vi "GDSError_LogErrorInformation.vi"(1 "State":string, 2 "LocalVariableData":variant, 3 "ExtraErrorInfo":string, 5 "error in (no error)":errorcluster) -> (19 "error out":errorcluster)   [LabVIEW 2016]
doc: "You can use this VI to generate errors."
uses:
  <resource>/Framework/Providers/Open_GDS/ClassProviders/Common/Error/GDSError_LogCluster.ctl
  <resource>/Framework/Providers/Open_GDS/ClassProviders/Common/Error/private/GDSError_LogCases.ctl
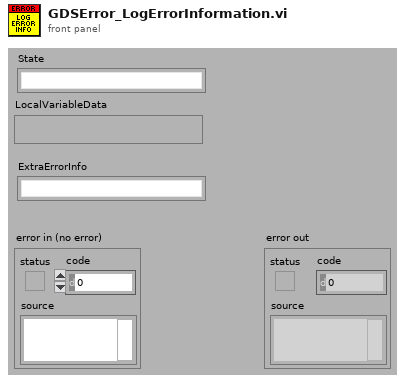
[diagram p1: front panel]
types:
  T1 = typedef "GDSError_LogCases.ctl" = enum16{"Init", "AddError", "ReadFirstError", "ReadLatestError", "ReadAllErrors", "ClearError", "ClearAllErrors"}
  T2 = typedef "GDSError_LogCluster.ctl" = cluster{"Time":timestamp, string, "error IO":errorcluster, "State":string, "LocalVariabelXML":string, "ExtraErrorInfo":string}
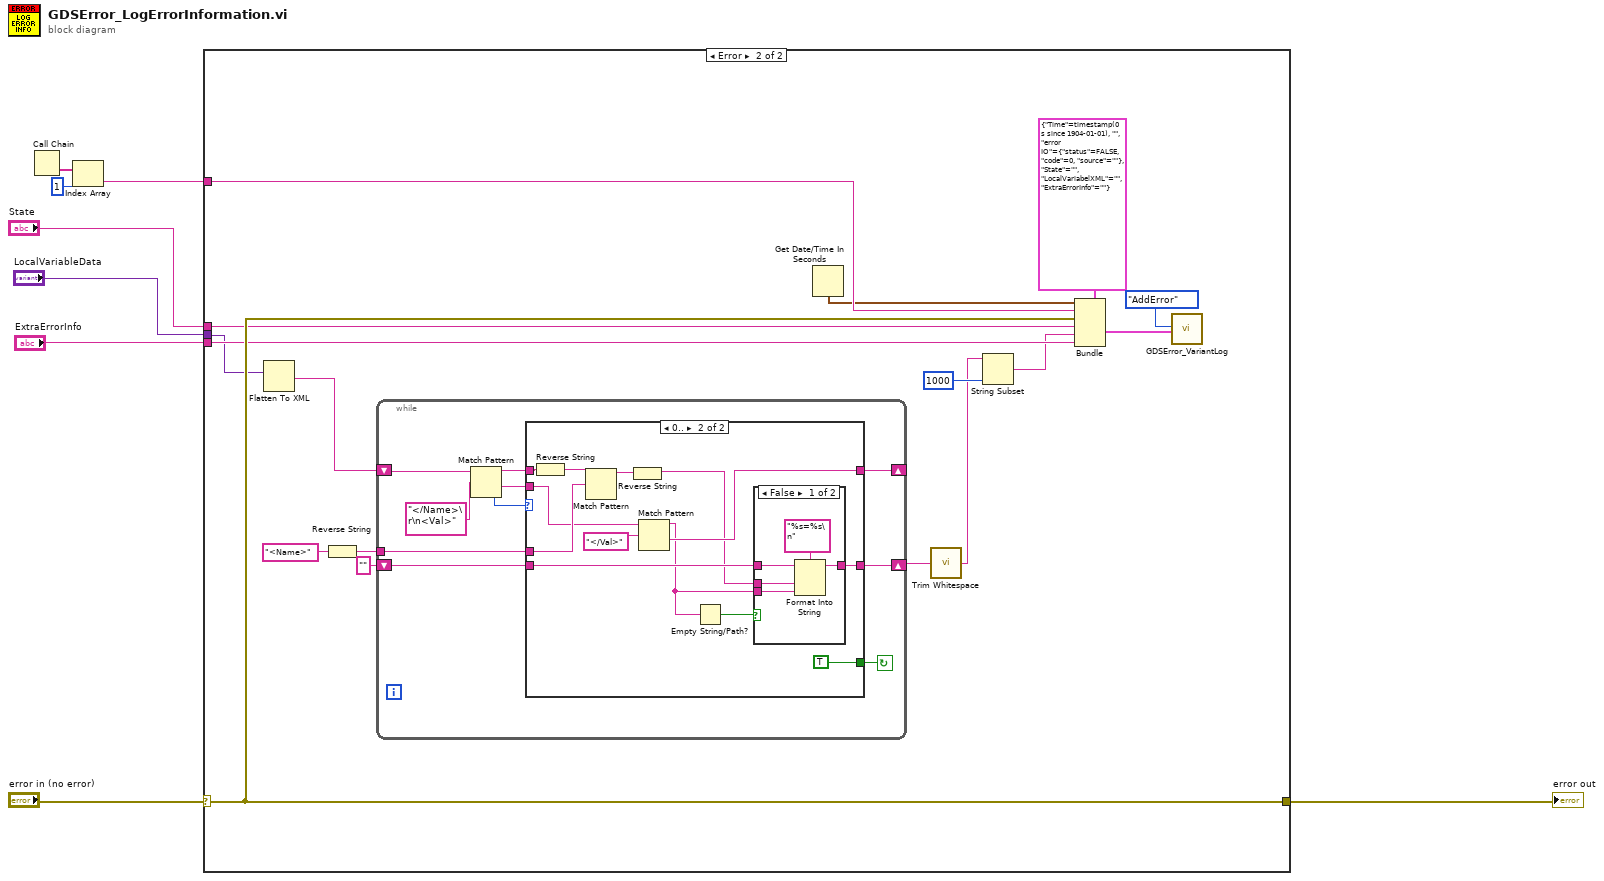
[diagram p0: block diagram]
diagram:
  n1 = Call Chain() -> (call chain=w5:string[])
  n2 = Index Array(array=w5, index=1) -> (element=w3:string)
  n3 = case shown="Error" "error in (no error)" {
    selector: "error in (no error)" -> [w9 w26]
    tunnel: [w9 w26] -> w7
    tunnel: "State" -> [_ w25]
    tunnel: w3 -> [_ w24]
    tunnel: "LocalVariableData" -> [_ w18]
    tunnel: "ExtraErrorInfo" -> [_ w23]
    frame No Error {
    }
    frame Error {
      n4 = Flatten To XML(anything=w18) -> (xml string=w11:string)
      n5 = Reverse String(1:"<Name>" ("regular expression")) -> (0:w14:string)
      n6 = while {
        shift-right: [w31] -> _
        shift-left: w11 -> [w36]
        tunnel: w14 -> [w33]
        shift-right: [w30] -> w12
        shift-left: "" -> [w29]
        stop <- w27 continue-if-true
        n7 = Match Pattern(string=w36, regular expression="</Name>\r\n<Val>") -> (before substring=w34:string, after substring=w32:string, offset past match=w28:i32)  [unwired: 1 in, 1 out]
        n8 = case shown="0.." w28 {
          tunnel: w34 -> [_ w50]
          tunnel: w33 -> [_ w48]
          tunnel: w32 -> [_ w46]
          tunnel: [_ w45] -> w31
          tunnel: [w37 w44] -> w30
          tunnel: w29 -> [w37 w43]
          tunnel: [_ TRUE] -> w27
          frame -1, Default {
          }
          frame 0.. {
            n9 = Reverse String(1:w50) -> (0:w49:string)
            n10 = Match Pattern(string=w49, regular expression=w48) -> (before substring=w47:string)  [unwired: 1 in, 3 out]
            n11 = Reverse String(1:w47) -> (0:w42:string)
            n12 = Match Pattern(string=w46, regular expression="</Val>") -> (before substring=w39:string, after substring=w45:string)  [unwired: 1 in, 2 out]
            n13 = Empty String/Path?(string/path=w39) -> (empty?=w38:bool)
            n14 = case shown="False" w38 {
              tunnel: [w54 w56] -> w44
              tunnel: w43 -> [w53 w56]
              tunnel: w42 -> [w52 _]
              tunnel: w39 -> [w51 _]
              frame False {
                n15 = Format Into String(format string="%s=%s\n", initial string=w53, w52, w51) -> (resulting string=w54:string)  [unwired: 1 in, 1 out]
              }
              frame True {
              }
            }
          }
        }
      }
      n16 = Get Date/Time In Seconds() -> (seconds since 1Jan1904=w19:timestamp)
      n17 = call <vilib>:"Trim Whitespace.vi"("string"=w12) -> ("trimmed string"=w10:string)  [unwired: 1 in]
      n18 = String Subset(string=w10, length (rest)=1000 ("y")) -> (substring=w16:string)  [unwired: 1 in]
      n19 = Bundle(cluster=T2 {"Time"=timestamp(0 s since 1904-01-01), "", "error IO"={"status"=FALSE, "code"=0, "source"=""}, "State"="", "LocalVariabelXML"="", "ExtraErrorInfo"=""} ("ErrorLogCluster"), "Time"=w19, w24, "error IO"=w26, "State"=w25, "LocalVariabelXML"=w16, "ExtraErrorInfo"=w23) -> (w21:T2)
      n20 = call <resource>:"GDSError_VariantLog.vi"("cases"=GDSError_LogCases."AddError", "VariantError"=w21) -> ()  [unwired: 16 in, 2 out]
    }
  }
  "error out" <- w7
